vi "Destroy.vi"(10 "Error":errorcluster, 11 "Destroy in":refnum<class "Destroy.lvclass">) -> (0 "error out":errorcluster, 3 "Destroy out":refnum<class "Destroy.lvclass">)   [LabVIEW 2021, in "Destroy.lvlib" / "Destroy.lvclass"]
uses:
  Destroy.lvclass
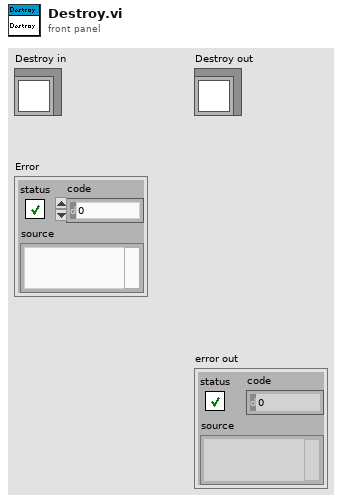
[diagram p1: front panel]
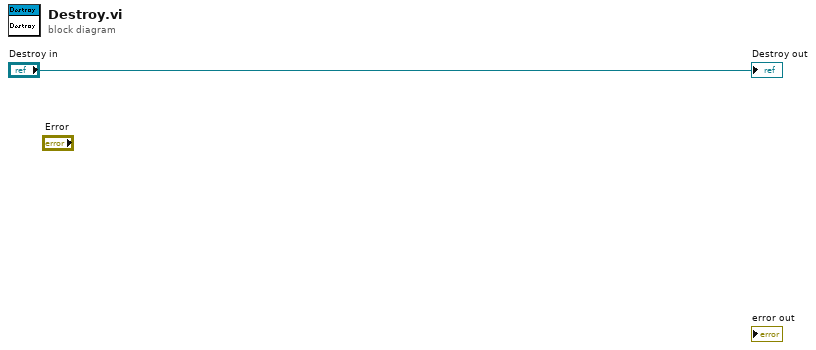
[diagram p0: block diagram]
diagram:
  "Destroy out" <- "Destroy in"
